vi "STD write.vi"(8 "error in (no error)":errorcluster, 10 "Message":string, 11 "STD IN/OUT":u32(ring)=4294967284 items=["STD_OUTPUT_HANDLE"=4294967285, "STD_ERROR_HANDLE"=4294967284]) -> (0 "error out":errorcluster, 3 "Bytes written":u32)   [LabVIEW 2012, in "Copy of LightPipes.lvlib"]
uses:
  Copy of LightPipes.lvlib
  kernel32.dll
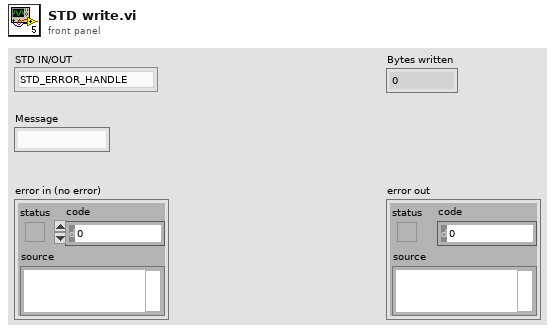
[diagram p1: front panel]
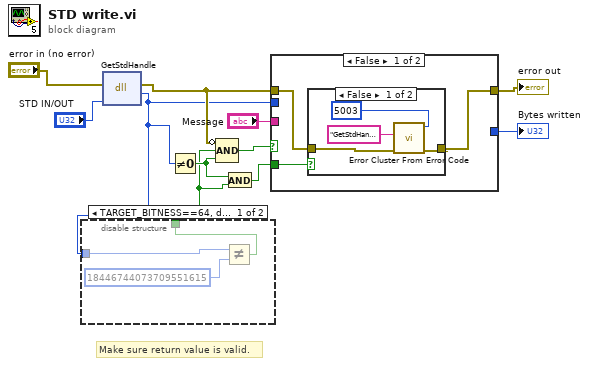
[diagram p0: block diagram]
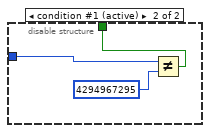
[diagram p2: hidden frame]
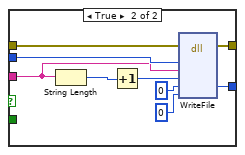
[diagram p4: hidden frame]
diagram:
  # "Make sure return value is valid."
  n1 = dll-call lib="kernel32.dll" fn="GetStdHandle"(error in="error in (no error)", "nStdHandle"="STD IN/OUT") -> (error out=w9:errorcluster, "HANDLE"=w4:u64)  [unwired: 3 in, 1 out]
  n2 = disable-structure shown="TARGET_BITNESS==64, default" {
    disable-tunnel: w4 -> [w14 w16]
    disable-tunnel: [w12 w15] -> w2
    frame condition #0 {
      n3 = Not Equal?(x=w14, y=u64 18446744073709551615) -> (x != y?=w12:bool)
    }
    frame condition #1 (active) {
      n4 = Not Equal?(x=w16, y=u64 4294967295) -> (x != y?=w15:bool)
    }
  }
  n5 = Not Equal To 0?(x=w4) -> (x != 0?=w3:bool)
  n6 = Compound Arithmetic op=AND(invert w9, w2, w3) -> (w8:bool)
  n7 = And(x=w3, y=w2) -> (x .and. y?=w1:bool)
  n8 = case shown="False" w8 {
    tunnel: w9 -> [w20 w34]
    tunnel: w4 -> [_ w33]
    tunnel: "Message" -> [_ w32]
    tunnel: [w19 w27] -> w6
    tunnel: [_ w26] -> w7
    tunnel: w1 -> [w18 _]
    frame False {
      n9 = case shown="False" w18 {
        tunnel: w20 -> [w24 w25]
        tunnel: [w21 w25] -> w19
        frame False {
          n10 = call <vilib>:"Error Cluster From Error Code.vi"("error in (no error)"=w24, "error message (\"\")"="GetStdHandle failed." ("error message (\"\")"), "error code (0)"=5003) -> ("error out"=w21:errorcluster)  [unwired: 6 in]
        }
        frame True {
        }
      }
    }
    frame True {
      n11 = String Length(string=w32) -> (length=w31:i32)
      n12 = Increment(x=w31) -> (x+1=w30:i32)
      n13 = dll-call lib="kernel32.dll" fn="WriteFile"(error in=w34, "hFile"=w33, "lpBuffer"=w32, "nNumberOfBytesToWrite"=w30, "lpNumberOfBytesWritten"=u32 0, "lpOverlapped"=u64 0) -> (error out=w27:errorcluster, "lpNumberOfBytesWritten"=w26:u32)  [unwired: 7 in, 1 out]
    }
  }
  "error out" <- w6
  "Bytes written" <- w7
